vi "determine Warnings(Challenge).vi"() -> ()   [LabVIEW 2014]
panel:
  in  "Current Temp 2":dbl
  in  "Min Temp 2":dbl
  out "Warning Text 2":string="Freeze Warning"
  out "Warning? 2":bool
  in  "Max Temp 2":dbl
  out "Warning Text":string="Freeze Warning"
  out "Warning?":bool
  in  "Min Temp":dbl
  in  "Max Temp":dbl
  in  "Current Temp":dbl
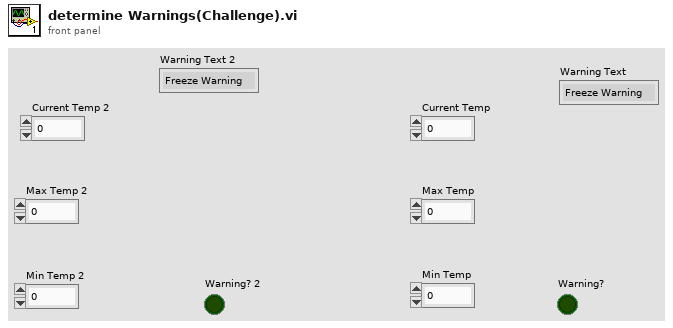
[diagram p1: front panel]
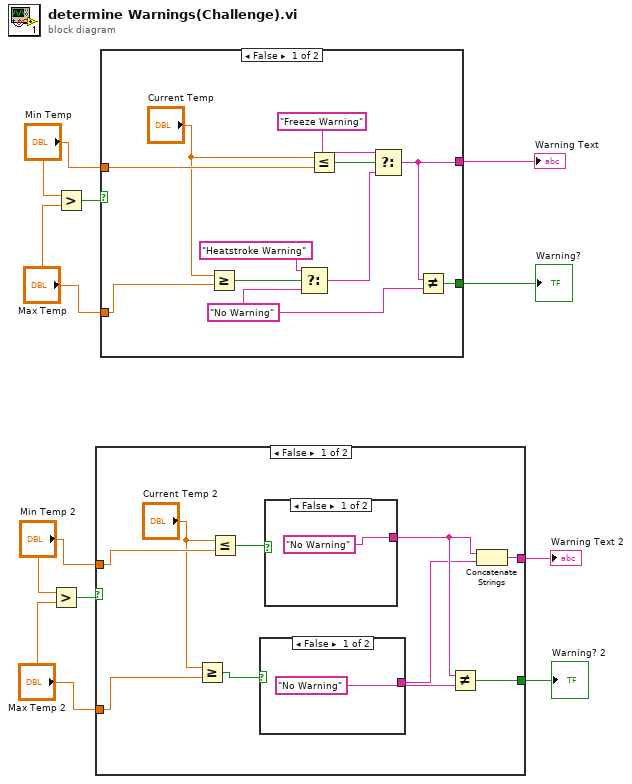
[diagram p0: block diagram]
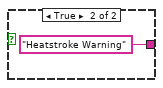
[diagram p2: hidden frame]
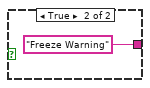
[diagram p3: hidden frame]
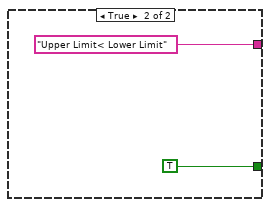
[diagram p4: hidden frame]
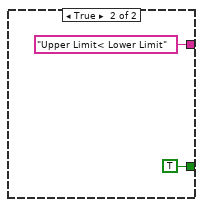
[diagram p5: hidden frame]
diagram:
  n1 = Greater?(x="Min Temp 2", y="Max Temp 2") -> (0:w3:bool)
  n2 = Greater?(x="Min Temp", y="Max Temp") -> (0:w8:bool)
  n3 = case shown="False" w3 {
    tunnel: [w13 "Upper Limit< Lower Limit" ("Warning Text")] -> w5
    tunnel: [w14 TRUE] -> w4
    tunnel: "Max Temp 2" -> [w16 _]
    tunnel: "Min Temp 2" -> [w19 _]
    frame False {
      n4 = Greater Or Equal?(x="Current Temp 2", y=w16) -> (x >= y?=w15:bool)
      n5 = Less Or Equal?(x="Current Temp 2", y=w19) -> (x <= y?=w18:bool)
      n6 = case shown="False" w15 {
        tunnel: ["No Warning" ("Warning Text") "Heatstroke Warning" ("Warning Text")] -> w11
        frame False {
        }
        frame True {
        }
      }
      n7 = case shown="False" w18 {
        tunnel: ["No Warning" ("Warning Text") "Freeze Warning" ("Warning Text")] -> w12
        frame False {
        }
        frame True {
        }
      }
      n8 = Not Equal?(x=w12, y=w11) -> (x != y?=w14:bool)
      n9 = Concatenate Strings(w12, w11) -> (w13:string)
    }
    frame True {
    }
  }
  "Warning? 2" <- w4
  "Warning Text 2" <- w5
  n10 = case shown="False" w8 {
    tunnel: [w30 "Upper Limit< Lower Limit" ("Warning Text")] -> w10
    tunnel: [w29 TRUE] -> w9
    tunnel: "Max Temp" -> [w28 _]
    tunnel: "Min Temp" -> [w27 _]
    frame False {
      w31 = "No Warning" ("Warning Text")
      n11 = Greater Or Equal?(x="Current Temp", y=w28) -> (x >= y?=w36:bool)
      n12 = Select(t="Heatstroke Warning" ("Warning Text"), s=w36, f=w31) -> (s? t:f=w32:string)
      n13 = Less Or Equal?(x="Current Temp", y=w27) -> (x <= y?=w34:bool)
      n14 = Select(t="Freeze Warning" ("Warning Text"), s=w34, f=w32) -> (s? t:f=w30:string)
      n15 = Not Equal?(x=w30, y=w31) -> (x != y?=w29:bool)
    }
    frame True {
    }
  }
  "Warning?" <- w9
  "Warning Text" <- w10
